vi "fix channel lists.vi"(7 "Type":T3, 8 "error in":errorcluster, 9 "channels in system definition":T2(array[cluster]) {"Channel Ref out" format="%.0x"}, 10 "cluster":variant, 11 "folder":T1 format="%.0x") -> (0 "error out":errorcluster)   [LabVIEW 2015, in "Scriptable Model Interface System Explorer.lvlib"]
uses:
  Scriptable Model Interface System Explorer.lvlib
  <vilib>/NI Veristand/Custom Device API/Custom Device Channel Type.ctl
  <vilib>/NI Veristand/Custom Device API/Custom Device Item Ref.ctl
  <vilib>/NI Veristand/Custom Device API/Custom Device Channel.ctl
  Shared/Scriptable Model Interface Shared.lvlib
  <vilib>/NI Veristand/Custom Device API/Custom Device API.lvlib
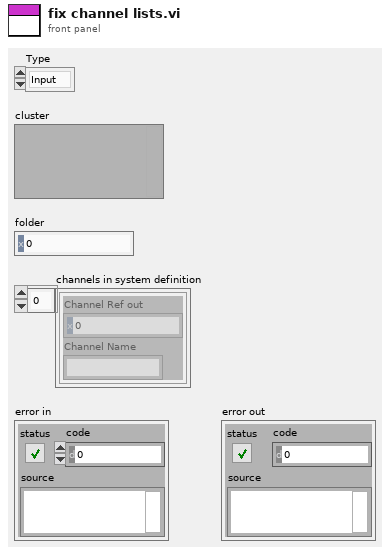
[diagram p1: front panel]
types:
  T1 = typedef "Custom Device API.lvlib/Custom Device Item Ref.ctl" = u64
  T2 = cluster{"Channel Ref out":T1, "Channel Name":string}[]
  T3 = typedef "Custom Device API.lvlib/Custom Device Channel Type.ctl" = enum16{"Input", "Output"}
  T4 = typedef "Scriptable Model Interface Shared.lvlib/channel id.ctl" = cluster{"Name":string, "index":i32}
  T5 = typedef "Custom Device API.lvlib/Custom Device Channel.ctl" = cluster{"Type":T3, "Units":string, "Default Value":dbl, "Faultable":bool, "Scalable":bool}
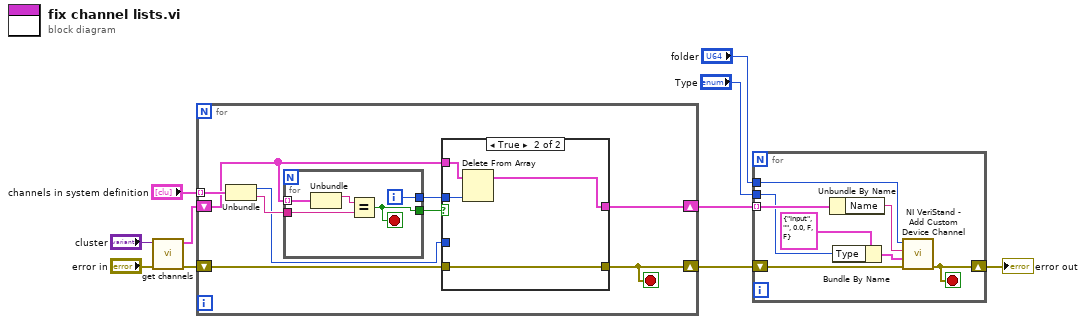
[diagram p0: block diagram]
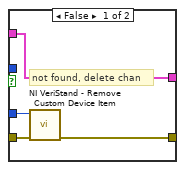
[diagram p2: hidden frame]
diagram:
  n1 = call "get channels.vi"("error in"="error in", "cluster in"="cluster") -> ("error out"=w4:errorcluster, "channels"=w3:T4[])  [unwired: 8 in]
  n2 = for {
    tunnel: "channels in system definition" -> [w19] mode=indexing
    shift-right: [w15] -> w5
    shift-left: w3 -> [w14]
    shift-right: [w12] -> w6
    shift-left: w4 -> [w16]
    stop <- w12 stop-if-true
    n3 = Unbundle(w19) -> ("Channel Ref out"=w11:T1, "Channel Name"=w18:string)
    n4 = for {
      tunnel: w14 -> [w32] mode=indexing
      tunnel: w18 -> [w30]
      tunnel: [w29] -> w13
      tunnel: [w28] -> w17
      i -> [w29]
      stop <- w28 stop-if-true
      n5 = Unbundle(w32) -> ("Name"=w31:string)  [unwired: 1 out]
      n6 = Equal?(x=w31, y=w30) -> (x = y?=w28:bool)
    }
    n7 = case shown="True" w17 {
      tunnel: w16 -> [w22 w24]
      tunnel: [w23 w26] -> w15
      tunnel: w14 -> [w23 w27]
      tunnel: w13 -> [_ w25]
      tunnel: [w21 w24] -> w12
      tunnel: w11 -> [w20 _]
      frame False {
        # "not found, delete chan"
        n8 = call <vilib>:"NI VeriStand - Remove Custom Device Item.vi"("error in (no error)"=w22, "Item Ref in"=w20) -> ("error out"=w21:errorcluster)  [unwired: 8 in, 1 out]
      }
      frame True {
        n9 = Delete From Array(array=w27, index=w25) -> (array with subset deleted=w26:T4[])  [unwired: 1 in, 1 out]
      }
    }
  }
  n10 = for {
    tunnel: w5 -> [w37] mode=indexing
    shift-right: [w39] -> w7
    shift-left: w6 -> [w40]
    tunnel: "folder" -> [w38]
    tunnel: "Type" -> [w33]
    stop <- w39 stop-if-true
    n11 = Unbundle By Name(w37) -> ("Name"=w36:string)
    n12 = Bundle By Name(cluster=T5 {"Type"=enum."Input", "Units"="", "Default Value"=0.0, "Faultable"=FALSE, "Scalable"=FALSE} ("Channel"), "Type"=w33) -> (w34:T5)
    n13 = call <vilib>:"NI VeriStand - Add Custom Device Channel.vi"("error in (no error)"=w40, "Channel"=w34, "Channel Name"=w36, "Parent Ref in"=w38) -> ("error out"=w39:errorcluster)  [unwired: 4 in, 3 out]
  }
  "error out" <- w7
